vi "fpga_transmission_control_3V4_VGA.vi"() -> ()   [LabVIEW 2017]
uses:
  Control 1.ctl
  <vilib>/Instr/_visa.llb/VISA Configure Serial Port (Serial Instr).vi
panel:
  out "PWM 2":bool
  out "Output":bool
  out "outcome":u32
  out "currentType":string
  out "Time":dbl(slide) scale=0.0..100.0
  out "Progress":dbl(slide) scale=0.0..100.0
  in  "error in (no error)":errorcluster
  out "PWM":bool
  out "pattern":u32
  in  "Timeslot":bool
  out "type":string
  out "Kombi Chart":cluster{u16, i16}(graph)
  out "contingency":string
  in  "Array":T2(array[cluster]) {"duration" step=1}
  out "Timeslot":i32
  out "Timer":dbl caption="Elapsed Time (s)"
  out "Sign":bool
  out "deleted portion":u8[](array[numeric])
  out "data":bool
  out "x-y":u16
  out "Error String":string
  out "error out":errorcluster
  out "Timing":u32
  out "Int_pixel":i16
  out "Pixel":u16(graph)
  out "AD_Value":i16
  in  "millisecond timer value 2":u32
  out "AD_Chart":i16(graph)
  in  "Path":path
  out "Read":bool
  in  "Stop Program":bool
  in  "Start":bool
  in  "VISA resource name":refnum<visa-resource-name>
  # "UR Elektronik Biologie\nTerminal V 3.4"
types:
  T1 = typedef "Control 1.ctl" = u32
  T2 = cluster{"type":string, "duration":T1, "outcome":u32, "pattern":u32, "coup_coeff":u32, "contingency":string}[]
  T3 = cluster{"String":string, i32, i32, u32, u32, "String":string}[]
  T4 = enum16{"Idel", "State1", "State2", "State3", "State4"}
  T5 = enum16{"open", "replace", "create", "open or create", "replace or create", "replace or create with confirmation"}
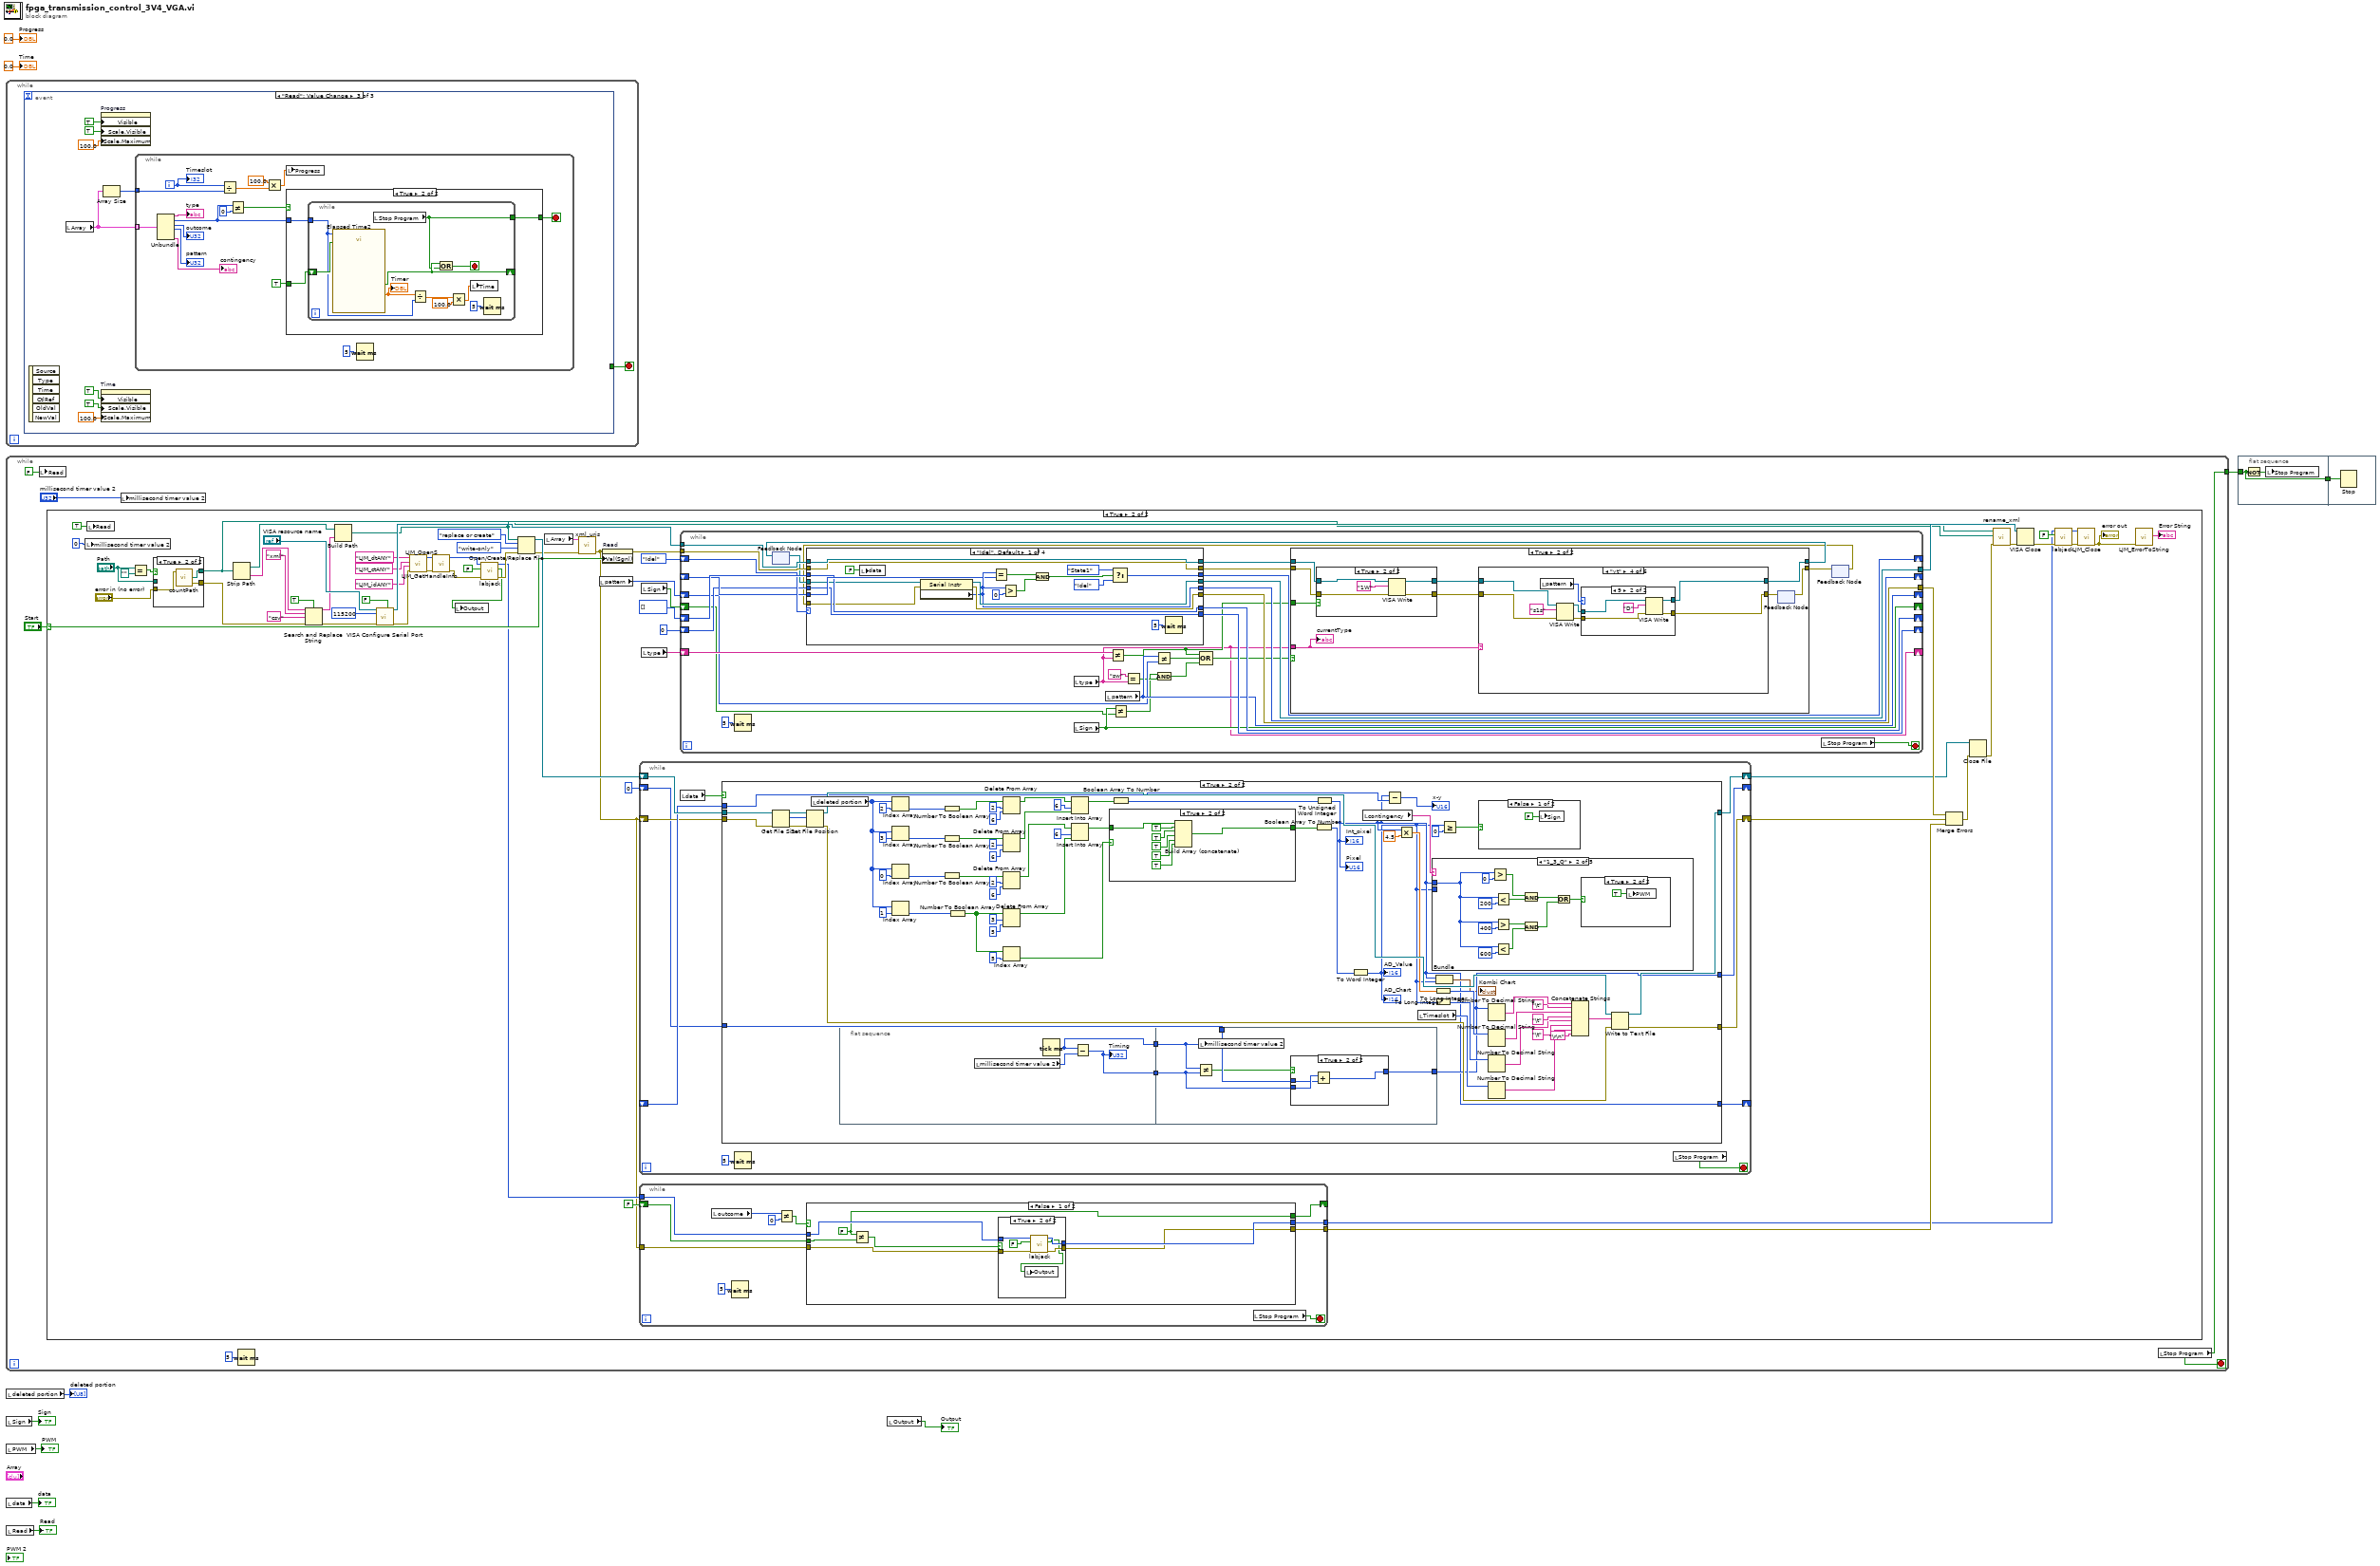
[diagram p0: block diagram]
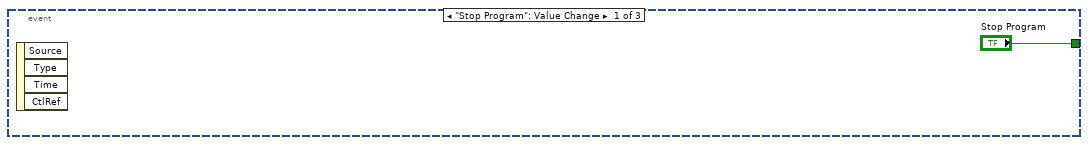
[diagram p2: hidden frame]
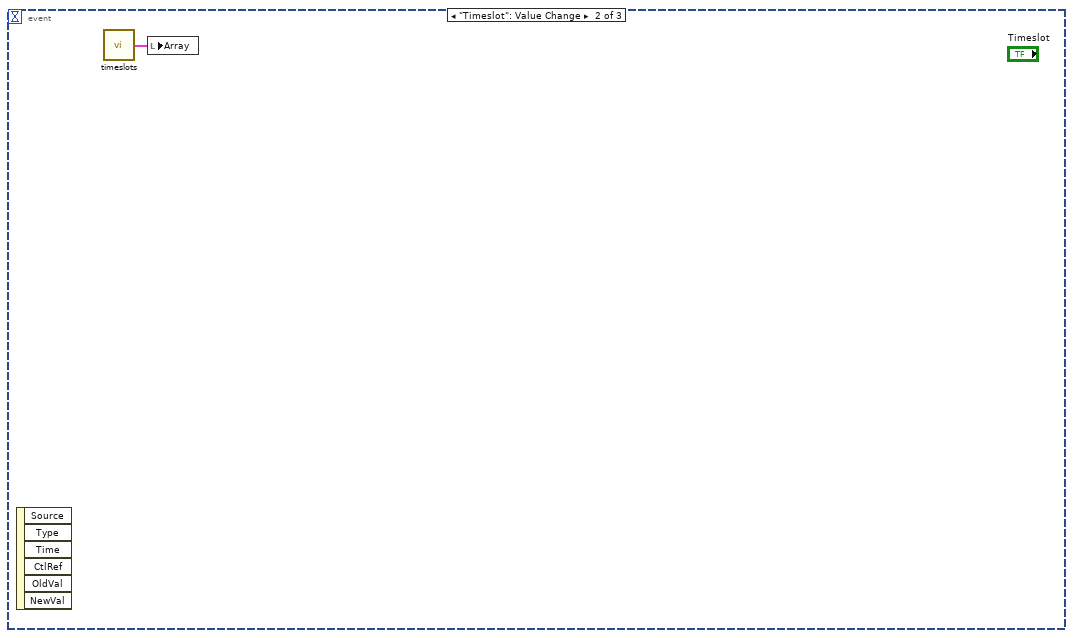
[diagram p3: hidden frame]
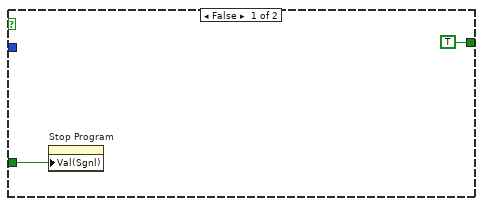
[diagram p4: hidden frame]
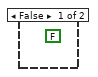
[diagram p5: hidden frame]
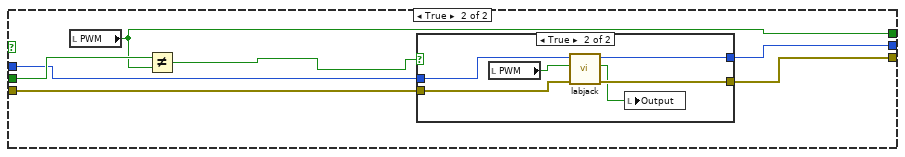
[diagram p8: hidden frame]
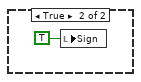
[diagram p11: hidden frame]
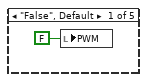
[diagram p12: hidden frame]
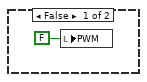
[diagram p13: hidden frame]
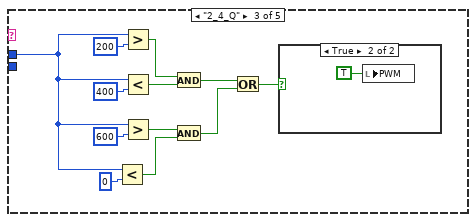
[diagram p14: hidden frame]
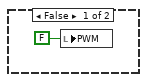
[diagram p15: hidden frame]
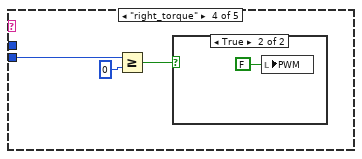
[diagram p16: hidden frame]
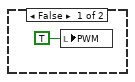
[diagram p17: hidden frame]
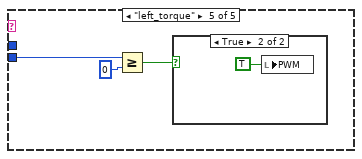
[diagram p18: hidden frame]
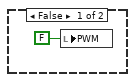
[diagram p19: hidden frame]
diagram:
  n1 = while {
    stop <- w11 stop-if-true
    n2 = event shown="[2] \"Read\": Value Change" {
      selector: _ -> [_ _ _]
      dyn-events: _ -> [_ _ _]
      timeout: _ -> [_ _ _]
      tunnel: ["Stop Program" _ _] -> w11
      event "Stop Program": Value Change {
        n3 = event-data() -> ()  [unwired: 1 in, 4 out]
      }
      event "Timeslot": Value Change {
        n4 = event-data() -> ()  [unwired: 1 in, 6 out]
        n5 = call "timeslots.vi"() -> ("array of clusters"=w13:T3)  [unwired: 2 in]
        n6 = local write "Array"(w13) -> ()
      }
      event "Read": Value Change {
        n7 = event-data() -> ()  [unwired: 1 in, 6 out]
        n8 = local read "Array"() -> (w21:T2)
        n9 = property on="Progress" class="Slide (strict)"("Visible"=TRUE, "Scale.Visible"=TRUE ("Visible"), "Scale.Maximum"=100.0 ("Scale.Range:Maximum")) -> ()  [unwired: 2 in, 2 out]
        n10 = property on="Time" class="Slide (strict)"("Visible"=TRUE, "Scale.Visible"=TRUE ("Visible"), "Scale.Maximum"=100.0 ("Scale.Range:Maximum")) -> ()  [unwired: 2 in, 2 out]
        n11 = Array Size(array=w21) -> (size(s)=w20:i32)
        n12 = while {
          tunnel: w21 -> [w35] mode=indexing
          tunnel: w20 -> [w27]
          i -> [w26]
          stop <- w37 stop-if-true
          n13 = Unbundle(w35) -> ("type"=→"type":string, "duration"=w32:T1, "outcome"=→"outcome":u32, "pattern"=→"pattern":u32, "contingency"=→"contingency":string)  [unwired: 1 out]
          n14 = Divide(x=w26, y=w27) -> (x/y=w25:dbl)
          n15 = Not Equal?(x=w32, y=u32 0) -> (x != y?=w33:bool)
          n16 = Multiply(x=100.0 ("y"), y=w25) -> (x*y=w23:dbl)
          n17 = local write "Progress"(w23) -> ()
          n18 = case shown="True" w33 {
            tunnel: w32 -> [_ w42]
            tunnel: [TRUE w41] -> w37
            tunnel: TRUE -> [w38 w40]
            frame False {
              n19 = property on="Stop Program" class="Bool (strict)"("Val(Sgnl)"=w38) -> ()  [unwired: 2 in, 2 out]
            }
            frame True {
              n20 = while {
                shift-right: [w51] -> _
                shift-left: w40 -> [w52]
                tunnel: [w49] -> w41
                tunnel: w42 -> [w44]
                stop <- w50 stop-if-true
                n21 = call "Elapsed Time2"("Time Target (s)"=w44, "Reset"=w52) -> ("Elapsed Time (s)"=w43:dbl, "Time has Elapsed"=w51:bool)  [unwired: 10 in, 6 out]
                "Timer" <- w43
                n22 = local read "Stop Program"() -> (w49:bool)
                n23 = Divide(x=w43, y=w44) -> (x/y=w47:dbl)
                n24 = Or(x=w51, y=w49) -> (x .or. y?=w50:bool)
                n25 = Multiply(x=w47, y=100.0) -> (x*y=w45:dbl)
                n26 = local write "Time"(w45) -> ()
                n27 = Wait (ms)(milliseconds to wait=u32 5) -> ()  [unwired: 1 out]
              }
            }
          }
          n28 = Wait (ms)(milliseconds to wait=u32 5) -> ()  [unwired: 1 out]
          "Timeslot" <- w26
        }
      }
    }
  }
  n29 = while {
    tunnel: [w56] -> w10
    stop <- w56 stop-if-true
    n30 = local write "Read"(FALSE) -> ()
    n31 = case shown="True" "Start" {
      selector: "Start" -> [_ w111]
      frame False {
        (unwired) FALSE
      }
      frame True {
        n32 = local write "millisecond timer value 2"(u32 0 ("millisecond timer value 2")) -> ()
        n33 = local write "Read"(TRUE) -> ()
        n34 = Equal?(x="Path", y=path "") -> (x = y?=w98:bool)
        n35 = case shown="True" w98 {
          tunnel: [w122 w125] -> w59
          tunnel: "Path" -> [w122 _]
          tunnel: [w121 w124] -> w70
          tunnel: "error in (no error)" -> [w121 w123]
          frame False {
          }
          frame True {
            n36 = call "countPath.vi"("error in (no error)"=w123) -> ("error out"=w124:errorcluster, "appended path"=w125:path)
          }
        }
        n37 = Strip Path(path=w59) -> (stripped path=w74:path, name=w73:string)
        n38 = Search and Replace String(case sensitive?=TRUE ("ignore case? (F)"), input string=w73, search string="xml", replace string="csv" ("replace string (\"\")"), error in=w70) -> (result string=w67:string, error out=w69:errorcluster)  [unwired: 3 in, 2 out]
        n39 = Build Path(base path=w74, name or relative path=w67) -> (appended path=w60:path)
        n40 = call-poly "VISA Configure Serial Port"("VISA resource name"="VISA resource name", "Enable Termination\nChar (T)"=FALSE ("Enable Termination\nChar (T)"), "baud rate (9600)"=u32 115200, "error in (no error)"=w69) -> ("VISA resource name out"=w93:refnum<visa-resource-name>, "error out"=w84:errorcluster)  [unwired: 10 in]
        n41 = call "LJM_OpenS.vi"("error in"=w84, "Identifier"="LJM_idANY", "ConnectionType"="LJM_ctANY", "DeviceType"="LJM_dtANY") -> ("error out"=w101:errorcluster, "Handle"=w100:i32)  [unwired: 6 in]
        n42 = call "LJM_GetHandleInfo.vi"("error in"=w101, "Handle In"=w100) -> ("error out"=w103:errorcluster, "Handle Out"=w102:i32)  [unwired: 2 in, 6 out]
        n43 = call "labjack.vi"("error out"=w103, "Boolean"=FALSE, "Handle Out"=w102) -> ("error out 2"=w106:errorcluster, "Boolean 2"=w58:bool, "Handle Out 2"=w105:i32)  [unwired: 6 in]
        n44 = local write "Output"(w58) -> ()
        n45 = Open/Create/Replace File(file path (use dialog)=w60, error in=w106, operation (0:open)=T5."replace or create", access (0:read/write)=enum16{"read/write", "read-only", "write-only"}."write-only") -> (refnum out=w77:refnum<file>, error out=w75:errorcluster)  [unwired: 2 in, 1 out]
        n46 = local read "Array"() -> (w76:T2)
        n47 = call "xml_uris.vi"("error in"=w75, "Array"=w76) -> ("error out"=w66:errorcluster)  [unwired: 2 in, 2 out]
        n48 = local read "pattern"() -> (w80:u32)
        n49 = property on="Read" class="Bool (strict)"(error in=w66, "Val(Sgnl)"=w111) -> (error out=w65:errorcluster)  [unwired: 1 in, 1 out]
        n50 = while {
          shift-right: [w176] -> w63
          shift-left: w77 -> [w177]
          shift-right: [w172] -> _
          shift-left: _ -> [w175]
          shift-right: [w171] -> w64
          shift-left: w66 -> [w170]
          shift-right: [w169] -> _
          shift-left: u32 0 -> [w168]
          stop <- w174 stop-if-true
          n51 = local read "data"() -> (w173:bool)
          n52 = case shown="True" w173 {
            tunnel: w170 -> [w181 w200]
            tunnel: [w181 w245] -> w171
            tunnel: w177 -> [w180 w206]
            tunnel: [w180 w244] -> w176
            tunnel: [w179 w183] -> w172
            tunnel: w175 -> [w179 w201]
            tunnel: [w178 w187] -> w169
            tunnel: w168 -> [w178 w188]
            frame False {
            }
            frame True {
              n53 = Get File Size(file=w206, error in=w200) -> (refnum out=w250:refnum<file>, size (in bytes)=w249:i64, 0:w248:errorcluster)
              n54 = Set File Position(offset (in bytes) (0)=w249, refnum=w250, error in=w248) -> (refnum out=w246:refnum<file>, error out=w247:errorcluster)  [unwired: 1 in]
              n55 = local read "deleted portion"() -> (w208:u8[])
              n56 = flat-sequence {
                tunnel: [w301] -> w243
                tunnel: [w300] -> w189
                tunnel: w243 -> [w304]
                tunnel: w189 -> [w305]
                tunnel: [w307] -> w187
                tunnel: w188 -> [w306]
                frame #0 {
                  n57 = local read "millisecond timer value 2"() -> (w302:u32)
                  n58 = Tick Count (ms)() -> (millisecond timer value=w301:u32)
                  n59 = Subtract(x=w301, y=w302) -> (x-y=w300:u32)
                  "Timing" <- w300
                }
                frame #1 {
                  n60 = Not Equal?(x=w304, y=w305) -> (x != y?=w303:bool)
                  n61 = local write "millisecond timer value 2"(w304) -> ()
                  n62 = case shown="True" w303 {
                    tunnel: w305 -> [_ w311]
                    tunnel: [u32 0 w310] -> w307
                    tunnel: w306 -> [_ w309]
                    frame False {
                    }
                    frame True {
                      n63 = Add(x=w311, y=w309) -> (x+y=w310:u32)
                    }
                  }
                }
              }
              n64 = Index Array(array=w208, index=2) -> (element=w203:u8)
              n65 = Index Array(array=w208, index=3) -> (element=w202:u8)
              n66 = Index Array(array=w208, index=0) -> (element=w205:u8)
              n67 = Index Array(array=w208, index=1) -> (element=w204:u8)
              n68 = Number To Boolean Array(number=w203) -> (Boolean array=w225:bool[])
              n69 = Number To Boolean Array(number=w202) -> (Boolean array=w228:bool[])
              n70 = Number To Boolean Array(number=w205) -> (Boolean array=w215:bool[])
              n71 = Number To Boolean Array(number=w204) -> (Boolean array=w234:bool[])
              n72 = Delete From Array(array=w225, length=2, index=6 ("length")) -> (array with subset deleted=w238:bool[])  [unwired: 1 out]
              n73 = Delete From Array(array=w228, length=2, index=6) -> (array with subset deleted=w239:bool[])  [unwired: 1 out]
              n74 = Delete From Array(array=w215, length=2, index=6 ("length")) -> (array with subset deleted=w218:bool[])  [unwired: 1 out]
              n75 = Delete From Array(array=w234, length=3, index=5) -> (array with subset deleted=w223:bool[])  [unwired: 1 out]
              n76 = Index Array(array=w234, index=5) -> (element=w236:bool)
              n77 = Insert Into Array(array=w238, index=6, new element=w239) -> (w232:bool[])
              n78 = Insert Into Array(array=w218, index=6, new element=w223) -> (w220:bool[])
              n79 = case shown="True" w236 {
                tunnel: w220 -> [w292 w299]
                tunnel: [w292 w294] -> w237
                frame False {
                }
                frame True {
                  n80 = Build Array (concatenate)(w299, TRUE ("new element/subarray"), TRUE ("new element/subarray"), TRUE ("new element/subarray"), TRUE ("new element/subarray"), TRUE ("element")) -> (w294:bool[])
                }
              }
              n81 = Boolean Array To Number(Boolean array=w232) -> (number=w233:u32)
              n82 = To Unsigned Word Integer(number=w233) -> (unsigned 16bit integer=w183:u16)
              "Pixel" <- w183
              "Int_pixel" <- w183
              n83 = Boolean Array To Number(Boolean array=w237) -> (number=w224:u32)
              n84 = To Word Integer(number=w224) -> (16bit integer=w182:i16)
              "AD_Chart" <- w182
              "AD_Value" <- w182
              n85 = local read "contingency"() -> (w190:string)
              n86 = Subtract(x=w183, y=w201) -> (x-y=→"x-y":u16)
              n87 = Multiply(x=w183, y=4.5) -> (x*y=w192:dbl)
              n88 = local read "Timeslot"() -> (w196:i32)
              n89 = case shown="\"1_3_Q\"" w190 {
                tunnel: w183 -> [_ w262 w276 _ _]
                tunnel: w182 -> [_ _ _ w282 w287]
                frame "False", Default {
                  n90 = local write "PWM"(FALSE ("pwm")) -> ()
                }
                frame "1_3_Q" {
                  n91 = Greater?(x=w262, y=u16 0 ("x")) -> (0:w257:bool)
                  n92 = Less?(x=w262, y=u16 200) -> (x < y?=w258:bool)
                  n93 = Greater?(x=w262, y=u16 400 ("a")) -> (0:w261:bool)
                  n94 = Less?(x=w262, y=u16 600 ("b")) -> (x < y?=w259:bool)
                  n95 = And(x=w257, y=w258) -> (x .and. y?=w256:bool)
                  n96 = And(x=w261, y=w259) -> (x .and. y?=w260:bool)
                  n97 = Or(x=w256, y=w260) -> (x .or. y?=w255:bool)
                  n98 = case shown="True" w255 {
                    frame False {
                      n99 = local write "PWM"(FALSE ("pwm")) -> ()
                    }
                    frame True {
                      n100 = local write "PWM"(TRUE ("pwm")) -> ()
                    }
                  }
                }
                frame "2_4_Q" {
                  n101 = Less?(x=w276, y=u16 0 ("b")) -> (x < y?=w273:bool)
                  n102 = Greater?(x=w276, y=u16 200 ("x")) -> (0:w271:bool)
                  n103 = Less?(x=w276, y=u16 400) -> (x < y?=w272:bool)
                  n104 = Greater?(x=w276, y=u16 600 ("a")) -> (0:w275:bool)
                  n105 = And(x=w271, y=w272) -> (x .and. y?=w270:bool)
                  n106 = And(x=w275, y=w273) -> (x .and. y?=w274:bool)
                  n107 = Or(x=w270, y=w274) -> (x .or. y?=w269:bool)
                  n108 = case shown="True" w269 {
                    frame False {
                      n109 = local write "PWM"(FALSE ("pwm")) -> ()
                    }
                    frame True {
                      n110 = local write "PWM"(TRUE ("pwm")) -> ()
                    }
                  }
                }
                frame "right_torque" {
                  n111 = Greater Or Equal?(x=w282, y=i16 0) -> (x >= y?=w283:bool)
                  n112 = case shown="True" w283 {
                    frame False {
                      n113 = local write "PWM"(TRUE ("pwm")) -> ()
                    }
                    frame True {
                      n114 = local write "PWM"(FALSE ("pwm")) -> ()
                    }
                  }
                }
                frame "left_torque" {
                  n115 = Greater Or Equal?(x=w287, y=i16 0) -> (x >= y?=w288:bool)
                  n116 = case shown="True" w288 {
                    frame False {
                      n117 = local write "PWM"(FALSE ("pwm")) -> ()
                    }
                    frame True {
                      n118 = local write "PWM"(TRUE ("pwm")) -> ()
                    }
                  }
                }
              }
              n119 = To Long Integer(number=w192) -> (32bit integer=w191:i32)
              n120 = To Long Integer(number=w182) -> (32bit integer=w194:i32)
              n121 = Bundle(w183, w182) -> (→"Kombi Chart":cluster{u16, i16})  [unwired: 1 in]
              n122 = Greater Or Equal?(x=w182, y=i16 0) -> (x >= y?=w184:bool)
              n123 = case shown="False" w184 {
                frame False {
                  n124 = local write "Sign"(FALSE) -> ()
                }
                frame True {
                  n125 = local write "Sign"(TRUE) -> ()
                }
              }
              n126 = Number To Decimal String(number=w187) -> (decimal integer string=w199:string)  [unwired: 1 in]
              n127 = Number To Decimal String(number=w191) -> (decimal integer string=w240:string)  [unwired: 1 in]
              n128 = Number To Decimal String(number=w194) -> (decimal integer string=w197:string)  [unwired: 1 in]
              n129 = Number To Decimal String(number=w196) -> (decimal integer string=w195:string)  [unwired: 1 in]
              n130 = Concatenate Strings(w199, "\t" ("string"), w240, "\t" ("string"), w197, "\t" ("string"), w195, "\r\n") -> (w207:string)
              n131 = Write to Text File(file (use dialog)=w246, text=w207, error in=w247) -> (refnum out=w244:refnum<file>, error out=w245:errorcluster)  [unwired: 1 in, 1 out]
            }
          }
          n132 = Wait (ms)(milliseconds to wait=u32 5) -> ()  [unwired: 1 out]
          n133 = local read "Stop Program"() -> (w174:bool)
        }
        n134 = while {
          tunnel: w105 -> [w134]
          tunnel: w66 -> [w133]
          shift-right: [w130] -> _
          shift-left: FALSE ("pwm") -> [w136]
          tunnel: [w132] -> w86
          tunnel: [w131] -> w113
          stop <- w135 stop-if-true
          n135 = local read "outcome"() -> (w129:u32)
          n136 = Wait (ms)(milliseconds to wait=u32 5) -> ()  [unwired: 1 out]
          n137 = Not Equal?(x=w129, y=u32 0) -> (x != y?=w127:bool)
          n138 = case shown="False" w127 {
            tunnel: w136 -> [w139 w158]
            tunnel: w134 -> [w143 w153]
            tunnel: w133 -> [w141 w154]
            tunnel: [w142 w157] -> w132
            tunnel: [w140 w156] -> w131
            tunnel: [w138 w155] -> w130
            frame False {
              w138 = FALSE ("Boolean")
              n139 = Not Equal?(x=w138, y=w139) -> (x != y?=w137:bool)
              n140 = case shown="True" w137 {
                tunnel: w143 -> [w145 w151]
                tunnel: [w145 w150] -> w142
                tunnel: w141 -> [w144 w149]
                tunnel: [w144 w148] -> w140
                frame False {
                }
                frame True {
                  n141 = call "labjack.vi"("error out"=w149, "Boolean"=FALSE, "Handle Out"=w151) -> ("error out 2"=w148:errorcluster, "Boolean 2"=w146:bool, "Handle Out 2"=w150:i32)  [unwired: 6 in]
                  n142 = local write "Output"(w146) -> ()
                }
              }
            }
            frame True {
              n143 = local read "PWM"() -> (w155:bool)
              n144 = Not Equal?(x=w158, y=w155) -> (x != y?=w152:bool)
              n145 = case shown="True" w152 {
                tunnel: w153 -> [w160 w166]
                tunnel: w154 -> [w159 w165]
                tunnel: [w160 w164] -> w157
                tunnel: [w159 w163] -> w156
                frame False {
                }
                frame True {
                  n146 = local read "PWM"() -> (w162:bool)
                  n147 = call "labjack.vi"("error out"=w165, "Boolean"=w162, "Handle Out"=w166) -> ("error out 2"=w163:errorcluster, "Boolean 2"=w161:bool, "Handle Out 2"=w164:i32)  [unwired: 6 in]
                  n148 = local write "Output"(w161) -> ()
                }
              }
            }
          }
          n149 = local read "Stop Program"() -> (w135:bool)
        }
        n150 = local read "Sign"() -> (w79:bool)
        n151 = local read "type"() -> (w107:string)
        n152 = while {
          tunnel: w93 -> [w344]
          tunnel: w65 -> [w343]
          shift-right: [w335] -> _
          shift-left: u8[] [] -> [w342]
          tunnel: [w341] -> w85
          tunnel: [w340] -> w118
          shift-right: [w339] -> _
          shift-left: T4."Idel" -> [w338]
          shift-right: [w337] -> _
          shift-left: _ -> [w336]
          shift-right: [w334] -> _
          shift-left: u8 0 -> [w333]
          shift-right: [w316] -> _
          shift-left: w107 -> [w327]
          shift-right: [w325] -> _
          shift-left: w80 -> [w324]
          shift-right: [w323] -> _
          shift-left: w79 -> [w322]
          stop <- w332 stop-if-true
          n153 = Wait (ms)(milliseconds to wait=u32 5) -> ()  [unwired: 1 out]
          n154 = feedback #1() -> (w330:refnum<visa-resource-name>)  [unwired: 1 in]
          n155 = local read "type"() -> (w316:string)
          n156 = local read "Sign"() -> (w323:bool)
          n157 = local read "pattern"() -> (w325:u32)
          n158 = Not Equal?(x=w327, y=w316) -> (x != y?=w317:bool)
          n159 = Not Equal?(x=w323, y=w322) -> (x != y?=w313:bool)
          n160 = Equal?(x="sw", y=w316) -> (x = y?=w314:bool)
          n161 = Not Equal?(x=w325, y=w324) -> (x != y?=w321:bool)
          n162 = And(x=w313, y=w314) -> (x .and. y?=w312:bool)
          n163 = Compound Arithmetic op=OR(w317, w321, w312) -> (w320:bool)
          n164 = local read "Stop Program"() -> (w332:bool)
          n165 = feedback #2() -> (w328:errorcluster)  [unwired: 1 in]
          n166 = case shown="\"Idel\", Default" w338 {
            tunnel: w344 -> [w460 w479 w499 w517]
            tunnel: w343 -> [w458 w477 w497 w514]
            tunnel: w342 -> [w463 w486 w502 w530]
            tunnel: [w471 w490 w498 w516] -> w341
            tunnel: [w470 w489 w496 w515] -> w340
            tunnel: [w473 w481 w503 w525] -> w339
            tunnel: [w469 w491 w501 w523] -> w337
            tunnel: w336 -> [w468 w492 w501 w523]
            tunnel: [w463 w485 w502 w529] -> w335
            tunnel: [w462 w480 w506 u8 0] -> w334
            tunnel: w333 -> [w462 w480 w504 w521]
            tunnel: [w460 w479 w499 w517] -> w318
            tunnel: w330 -> [w459 w478 w498 w516]
            tunnel: [w458 w477 w497 w514] -> w319
            tunnel: w328 -> [w457 w476 w496 w515]
            frame "Idel", Default {
              n167 = local write "data"(FALSE ("data")) -> ()
              n168 = property class="Serial Instr"(reference=w459, error in=w457) -> (reference out=w471:refnum<visa-resource-name>, error out=w470:errorcluster, "Serial Settings:Number of Bytes at Serial Port"=w469:u32)
              n169 = Equal?(x=w469, y=w468) -> (x = y?=w467:bool)
              n170 = Greater?(x=w469, y=u8 0) -> (0:w466:bool)
              n171 = And(x=w467, y=w466) -> (x .and. y?=w464:bool)
              n172 = Select(t=T4."State1", s=w464, f=T4."Idel") -> (s? t:f=w473:T4)
              n173 = Wait (ms)(milliseconds to wait=u32 5) -> ()  [unwired: 1 out]
            }
            frame "State1" {
              n174 = Array Size(array=w486) -> (size(s)=w488:i32)
              n175 = VISA Read(VISA resource name=w478, byte count=w492, error in (no error)=w476) -> (VISA resource name out=w490:refnum<visa-resource-name>, read buffer=w493:string, return count=w491:u32, error out=w489:errorcluster)
              n176 = String To Byte Array(string=w493) -> (unsigned byte array=w487:u8[])
              n177 = Insert Into Array(array=w486, index=w488, new element=w487) -> (w485:u8[])
              n178 = Array Size(array=w485) -> (size(s)=w483:i32)
              n179 = Greater?(x=w483, y=8) -> (0:w482:bool)
              n180 = Select(t=T4."State2", s=w482, f=T4."State1") -> (s? t:f=w481:T4)
            }
            frame "State2" {
              n181 = Index Array(array=w502, index=w504) -> (element=w510:u8)
              n182 = local write "data"(FALSE) -> ()
              n183 = And(x=w510, y=u8 192) -> (x .and. y?=w511:u8)
              n184 = Equal?(x=u8 0, y=w511) -> (x = y?=w507:bool)
              n185 = Select(t=T4."State3", s=w507, f=T4."State2") -> (s? t:f=w503:T4)
              n186 = Add(x=w504, y=u8 1) -> (x+y=w506:u8)
            }
            frame "State3" {
              n187 = Subtract(x=w521, y=u8 1) -> (x-y=w520:u8)
              n188 = local write "data"(TRUE ("data")) -> ()
              n189 = Delete From Array(array=w530, length=4, index=w520) -> (deleted portion=w522:u8[], array with subset deleted=w529:u8[])
              n190 = local write "deleted portion"(w522) -> ()
              n191 = Array Size(array=w529) -> (size(s)=w528:i32)
              n192 = Greater?(x=w528, y=8) -> (0:w526:bool)
              n193 = Select(t=T4."State2", s=w526, f=T4."Idel") -> (s? t:f=w525:T4)
            }
          }
          n194 = case shown="True" w320 {
            tunnel: w318 -> [w346 w350]
            tunnel: [w346 w353] -> w331
            tunnel: w319 -> [w345 w349]
            tunnel: [w345 w354] -> w329
            tunnel: w316 -> [_ w347]
            tunnel: w317 -> [_ w348]
            frame False {
            }
            frame True {
              n195 = case shown="True" w348 {
                tunnel: [w356 w362] -> w352
                tunnel: [w357 w361] -> w351
                tunnel: w350 -> [w357 w359]
                tunnel: w349 -> [w356 w358]
                frame False {
                }
                frame True {
                  n196 = VISA Write(VISA resource name=w359, write buffer="1W", error in (no error)=w358) -> (VISA resource name out=w361:refnum<visa-resource-name>, error out=w362:errorcluster)  [unwired: 1 out]
                }
              }
              n197 = case shown="\"yt\"" w347 {
                tunnel: w351 -> [w364 w371 w376 w384 w395 w432]
                tunnel: [w366 w370 w375 w378 w394 w431] -> w353
                tunnel: w352 -> [w363 w369 w374 w383 w397 w434]
                tunnel: [w365 w368 w373 w379 w396 w433] -> w355
                frame "False", Default {
                  n198 = VISA Write(VISA resource name=w364, write buffer="s4s", error in (no error)=w363) -> (VISA resource name out=w366:refnum<visa-resource-name>, error out=w365:errorcluster)  [unwired: 1 out]
                }
                frame "optomotorR" {
                  n199 = VISA Write(VISA resource name=w371, write buffer="s3r", error in (no error)=w369) -> (VISA resource name out=w370:refnum<visa-resource-name>, error out=w368:errorcluster)  [unwired: 1 out]
                }
                frame "optomotorL" {
                  n200 = VISA Write(VISA resource name=w376, write buffer="s3l", error in (no error)=w374) -> (VISA resource name out=w375:refnum<visa-resource-name>, error out=w373:errorcluster)  [unwired: 1 out]
                }
                frame "yt" {
                  n201 = local read "pattern"() -> (w382:u32)
                  n202 = VISA Write(VISA resource name=w384, write buffer="s1s", error in (no error)=w383) -> (VISA resource name out=w381:refnum<visa-resource-name>, error out=w380:errorcluster)  [unwired: 1 out]
                  n203 = case shown="9" w382 {
                    tunnel: w381 -> [w387 w391]
                    tunnel: w380 -> [w386 w390]
                    tunnel: [w386 w389] -> w379
                    tunnel: [w387 w388] -> w378
                    frame 0, Default {
                    }
                    frame 9 {
                      n204 = VISA Write(VISA resource name=w391, write buffer="D", error in (no error)=w390) -> (VISA resource name out=w388:refnum<visa-resource-name>, error out=w389:errorcluster)  [unwired: 1 out]
                    }
                  }
                }
                frame "sw" {
                  n205 = local read "pattern"() -> (w393:u32)
                  n206 = case shown="7" w393 {
                    tunnel: w397 -> [w398 w403 w419]
                    tunnel: [w398 w401 w418] -> w396
                    tunnel: w395 -> [w399 w404 w417]
                    tunnel: [w399 w402 w416] -> w394
                    frame 0, Default {
                    }
                    frame 8 {
                      n207 = local read "Sign"() -> (w400:bool)
                      n208 = case shown="False" w400 {
                        tunnel: w403 -> [w406 w413]
                        tunnel: [w405 w412] -> w401
                        tunnel: w404 -> [w408 w411]
                        tunnel: [w407 w410] -> w402
                        frame True {
                          n209 = VISA Write(VISA resource name=w408, write buffer="G", error in (no error)=w406) -> (VISA resource name out=w407:refnum<visa-resource-name>, error out=w405:errorcluster)  [unwired: 1 out]
                        }
                        frame False {
                          n210 = VISA Write(VISA resource name=w411, write buffer="B", error in (no error)=w413) -> (VISA resource name out=w410:refnum<visa-resource-name>, error out=w412:errorcluster)  [unwired: 1 out]
                        }
                      }
                    }
                    frame 7 {
                      n211 = local read "Sign"() -> (w415:bool)
                      n212 = case shown="True" w415 {
                        tunnel: w419 -> [w421 w428]
                        tunnel: [w420 w427] -> w418
                        tunnel: w417 -> [w423 w426]
                        tunnel: [w422 w425] -> w416
                        frame False {
                          n213 = VISA Write(VISA resource name=w423, write buffer="G", error in (no error)=w421) -> (VISA resource name out=w422:refnum<visa-resource-name>, error out=w420:errorcluster)  [unwired: 1 out]
                        }
                        frame True {
                          n214 = VISA Write(VISA resource name=w426, write buffer="B", error in (no error)=w428) -> (VISA resource name out=w425:refnum<visa-resource-name>, error out=w427:errorcluster)  [unwired: 1 out]
                        }
                      }
                    }
                  }
                }
                frame "fs" {
                  n215 = local read "pattern"() -> (w430:u32)
                  n216 = case shown="4" w430 {
                    tunnel: w434 -> [w435 w441 w446 w451 w456]
                    tunnel: [w435 w439 w444 w449 w454] -> w433
                    tunnel: w432 -> [w436 w440 w445 w450 w455]
                    tunnel: [w436 w438 w443 w448 w453] -> w431
                    frame 0, Default {
                    }
                    frame 3 {
                      n217 = VISA Write(VISA resource name=w440, write buffer="s3s", error in (no error)=w441) -> (VISA resource name out=w438:refnum<visa-resource-name>, error out=w439:errorcluster)  [unwired: 1 out]
                    }
                    frame 2 {
                      n218 = VISA Write(VISA resource name=w445, write buffer="s2s", error in (no error)=w446) -> (VISA resource name out=w443:refnum<visa-resource-name>, error out=w444:errorcluster)  [unwired: 1 out]
                    }
                    frame 1 {
                      n219 = VISA Write(VISA resource name=w450, write buffer="s1s", error in (no error)=w451) -> (VISA resource name out=w448:refnum<visa-resource-name>, error out=w449:errorcluster)  [unwired: 1 out]
                    }
                    frame 4 {
                      n220 = VISA Write(VISA resource name=w455, write buffer="s4s", error in (no error)=w456) -> (VISA resource name out=w453:refnum<visa-resource-name>, error out=w454:errorcluster)  [unwired: 1 out]
                    }
                  }
                }
              }
              n221 = feedback #3() -> (w354:errorcluster)  [unwired: 1 in]
              n222 = feedback-in #3(w355) -> ()
              "currentType" <- w347
            }
          }
          n223 = feedback-in #1(w331) -> ()
          n224 = feedback-in #2(w329) -> ()
        }
        n225 = Merge Errors(w118, w64, w113) -> (w117:errorcluster)
        n226 = Close File(refnum=w63, error in=w117) -> (error out=w62:errorcluster)  [unwired: 1 out]
        n227 = call "rename_xml.vi"("error in"=w62, "xml"=w59, "csv"=w60) -> ("error out"=w61:errorcluster)  [unwired: 4 in]
        n228 = VISA Close(VISA resource name=w85, error in (no error)=w61) -> (error out=w91:errorcluster)
        n229 = call "labjack.vi"("error out"=w91, "Boolean"=FALSE, "Handle Out"=w86) -> ("error out 2"=w92:errorcluster, "Handle Out 2"=w90:i32)  [unwired: 6 in, 1 out]
        n230 = call "LJM_Close.vi"("error in"=w92, "Handle"=w90) -> ("error out"=w89:errorcluster)  [unwired: 9 in]
        "error out" <- w89
        n231 = call "LJM_ErrorToString.vi"("error in"=w89) -> ("String"=→"Error String":string)  [unwired: 10 in]
      }
    }
    n232 = local write "millisecond timer value 2"("millisecond timer value 2") -> ()
    n233 = Wait (ms)(milliseconds to wait=u32 5) -> ()  [unwired: 1 out]
    n234 = local read "Stop Program"() -> (w56:bool)
  }
  n235 = local read "deleted portion"() -> (→"deleted portion":u8[])
  n236 = local read "Sign"() -> (→"Sign":bool)
  n237 = local read "PWM"() -> (→"PWM":bool)
  n238 = local read "data"() -> (→"data":bool)
  n239 = local read "Read"() -> (→"Read":bool)
  n240 = local read "Output"() -> (→"Output":bool)
  n241 = flat-sequence {
    tunnel: w10 -> [w535]
    tunnel: [w535] -> w9
    tunnel: w9 -> [w536]
    frame #0 {
      n242 = Not(x=w535) -> (.not. x?=w534:bool)
      n243 = local write "Stop Program"(w534) -> ()
    }
    frame #1 {
      n244 = Stop(stop? (T)=w536) -> ()
    }
  }
  "Progress" <- 0.0 ("Slide")
  "Time" <- 0.0 ("Progress 2")
